vi "Summary.vi"(8 "error in":errorcluster, 10 "depth":i32, 11 "node self ref":T1) -> (0 "error out":errorcluster, 2 "summary":T2[](array[typedef]))   [LabVIEW 2013, in "NISE_CEF_TreeControl.lvlib"]
doc: "Gets the summary of a node and all the subnodes. This descritpion can be used to update the tree control"
uses:
  NISE_CEF_TreeControl.lvlib
  Node/Summary.ctl
  Node/NodeRef.ctl
  Node/NISE_CEF_Node.lvclass
  Node/NISE_CEF_Node.lvclass/NISE_CEF_Node.ctl
  Node/ReadParent.vi
  Node/ReadChildren.vi
  Node/ReadNodeClass.vi
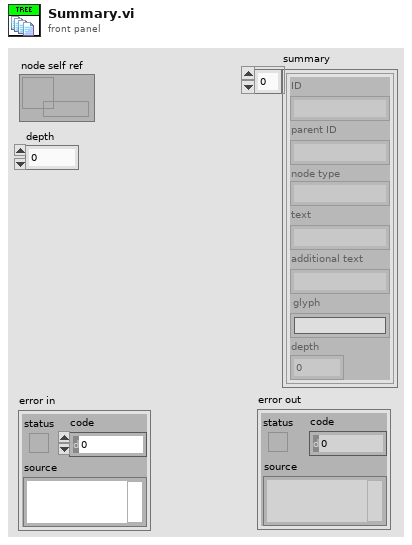
[diagram p1: front panel]
types:
  T1 = typedef "NISE_CEF_Node.lvclass/NodeRef.ctl" = refnum<data-value>
  T2 = typedef "NISE_CEF_Node.lvclass/Summary.ctl" = cluster{"ID":string, "parent ID":string, "node type":string, "text":string, "additional text":string, "glyph":string, "depth":i32}
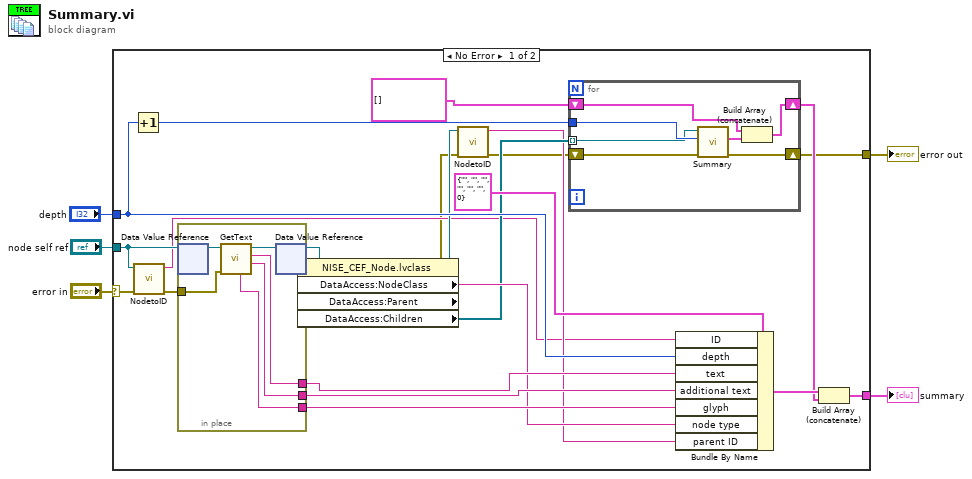
[diagram p0: block diagram]
diagram:
  n1 = case shown="No Error" "error in" {
    selector: "error in" -> [w12 w42]
    tunnel: [w6 w42] -> w4
    tunnel: "node self ref" -> [w14 _]
    tunnel: "depth" -> [w28 _]
    tunnel: [w27 _] -> w1
    frame No Error {
      n2 = Increment(x=w28) -> (x+1=w21:i32)
      n3 = call "NodetoID.vi"("error in"=w12, "node ref"=w14) -> ("error out"=w11:errorcluster, "ID"=w13:string)  [unwired: 8 in]
      n4 = in-place {
        in-place-border: [w34] -> w25
        in-place-border: [w33] -> w24
        in-place-border: [w32] -> w23
        in-place-border: w11 -> [w31]
        n5 = in-place-dvr #1(w14) -> (w30:refnum<class "NISE_CEF_Node.lvclass">)  [unwired: 1 out]
        n6 = call-dynamic "GetText.vi"("error in"=w31, "node in"=w30) -> ("additional text"=w34:string, "text"=w33:string, "node out"=w29:refnum<class "NISE_CEF_Node.lvclass">, "glyph"=w32:string)  [unwired: 5 in, 1 out]
        n7 = in-place-dvr #1(w29) -> (w10:T1, w9:errorcluster)
      }
      n8 = property class="NISE_CEF_Node.lvclass"(reference=w10, error in=w9) -> (error out=w8:errorcluster, "DataAccess:NodeClass"=w22:string, "DataAccess:Parent"=w16:T1, "DataAccess:Children"=w17:T1[])  [unwired: 1 out]
      n9 = call "NodetoID.vi"("error in"=w8, "node ref"=w16) -> ("error out"=w7:errorcluster, "ID"=w15:string)  [unwired: 8 in]
      n10 = for {
        tunnel: w17 -> [w37] mode=indexing
        tunnel: w21 -> [w41]
        shift-right: [w39] -> w18
        shift-left: T2[] [] ("childrensummary") -> [w40]
        shift-right: [w35] -> w6
        shift-left: w7 -> [w36]
        n11 = call "Summary.vi"("error in"=w36, "depth"=w41, "node self ref"=w37) -> ("error out"=w35:errorcluster, "summary"=w38:T2[])  [unwired: 7 in]
        n12 = Build Array (concatenate)(w40, w38) -> (w39:T2[])
      }
      n13 = Bundle By Name(cluster=T2 {"ID"="", "parent ID"="", "node type"="", "text"="", "additional text"="", "glyph"="", "depth"=0} ("nodeSummary"), "ID"=w13, "depth"=w28, "text"=w24, "additional text"=w25, "glyph"=w23, "node type"=w22, "parent ID"=w15) -> (w19:T2)
      n14 = Build Array (concatenate)(w19, w18) -> (w27:T2[])
    }
    frame Error {
    }
  }
  "error out" <- w4
  "summary" <- w1
